vi "Transform error.vi"(8 "error in (no error)":errorcluster, 9 "server errors":u8[](array[numeric]), 10 "return code":u8, 11 "client in":refnum<class "PuTTY Client.lvclass">) -> (0 "error out":errorcluster, 1 "server errors out":u8[](array[numeric]), 2 "return code out":u8, 3 "client out":refnum<class "PuTTY Client.lvclass">)   [LabVIEW 2020, in "NI_SSH.lvlib" / "PuTTY Client.lvclass"]
uses:
  <vilib>/net/SSH/Client/PuTTY/PuTTY Client.lvclass
  <vilib>/net/SSH/Client/Generic/Stderr Match Patterns.ctl
  <vilib>/net/SSH/Client/Generic/Generic Client.lvclass
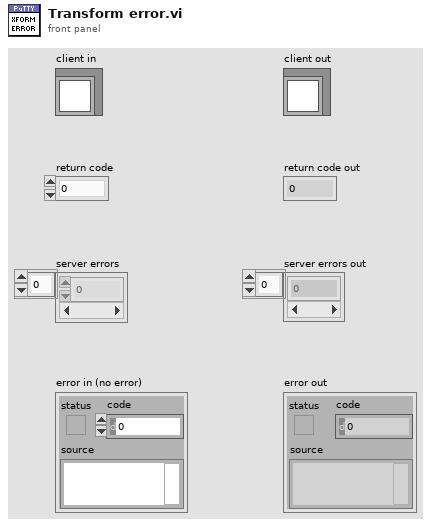
[diagram p1: front panel]
types:
  T1 = typedef "NI_SSH.lvlib/Generic Client.lvclass/Stderr Match Patterns.ctl" = cluster{"incorrect pubkey":string, "unknown pubkey":string, "crypto disallowed":string, "dns spoofing":string, "access denied":string}
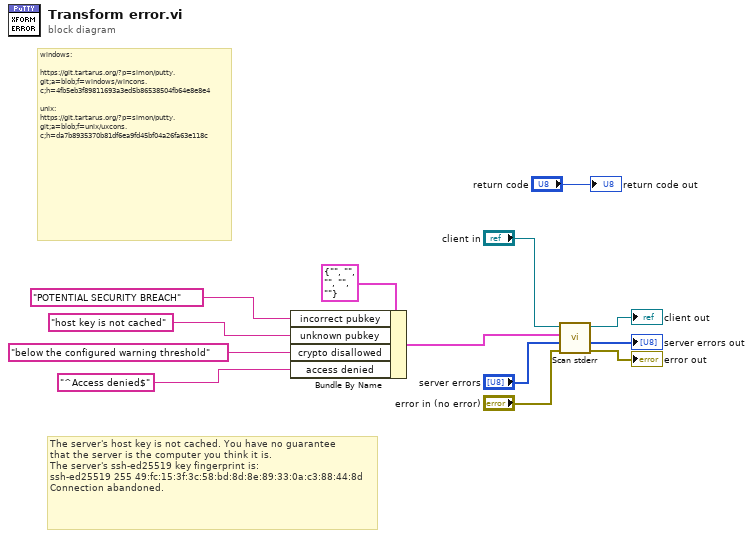
[diagram p0: block diagram]
diagram:
  # "windows:\n\nhttps://git.tartarus.org/?p=simon/putty.git;a=blob;f=windows/wincons.c;h=4fb5eb3f89811693a3ed5b86538504fb64e8e8e4\n\nunix:\nhttps://git.tartarus.org/?p=simon/putty.git;a=blob;f=unix/uxcons.c;h=da7b8935370b81df6ea9fd45bf04a26fa63e118c"
  # "The server's host key is not cached. You have no guarantee\nthat the server is the computer you think it is.\nThe server's ssh-ed25519 key fingerprint is:\nssh-ed25519 255 49:fc:15:3f:3c:58:bd:8d:8e:89:33:0a:c3:88:44:8d\nConnection abandoned."
  n1 = Bundle By Name(cluster=T1 {"incorrect pubkey"="", "unknown pubkey"="", "crypto disallowed"="", "dns spoofing"="", "access denied"=""} ("patterns"), "incorrect pubkey"="POTENTIAL SECURITY BREACH" ("regular expression"), "unknown pubkey"="host key is not cached" ("regular expression"), "crypto disallowed"="below the configured warning threshold" ("regular expression"), "access denied"="^Access denied$") -> (w6:T1)
  n2 = call-dynamic "Scan stderr.vi"("error in (no error)"="error in (no error)", "stderr in"="server errors", "patterns"=w6, "client in"="client in") -> ("error out"=→"error out":errorcluster, "stderr out"=→"server errors out":u8[], "client out"=→"client out":refnum<class "PuTTY Client.lvclass">)  [unwired: 5 in]
  "return code out" <- "return code"
